vi "MagPhasePlot.vi"(7 "PlotSource":T1, 8 "error in (no error)":errorcluster, 11 "AllData":T3 {"FlukeData"."DataAnalysisArray"."TimeStamp" format="%^<%.3X\n%x>T"; "FlukeData"."ModelDataArray"."FREQUENCY" format="%#_6f"; "FlukeData"."ModelDataArray"."TimeStamp" format="%^<%.3X\n%x>T"; "FlukeData"."PMUDataArray"."FREQUENCY" format="%#_6f"; "FlukeData"."PMUDataArray"."TimeStamp" format="%^<%.3X\n%x>T"; "NISTData"."DataAnlysisArray"."Time" format="%.6f"; "NISTData"."DataAnlysisArray"."TimeStamp" format="%^<%.3X\n%x>T"; "NISTData"."DUTDataArray"."TimeStamp" format="%^<%.3X\n%x>T"; "NISTData"."DUTDataArray"."Time" format="%.6f"; "NISTData"."NIDataArray"."TimeStamp" format="%^<%.3X\n%x>T"; "NISTData"."NIDataArray"."Time" format="%.6f"}) -> (0 "error out":errorcluster, 1 "Phase Plot":T2(graph), 2 "Mag Plot":T2(graph))   [LabVIEW 2014]
uses:
  typedefs/Alldata.ctl
  typedefs/NISTData.ctl
  typedefs/NIDataArray.ctl
  typedefs/NIData.ctl
  typedefs/PhasorRectangular.ctl
  typedefs/DUTData.ctl
  typedefs/NICalcAnalysis.ctl
  typedefs/CalcPhasorError.ctl
  typedefs/PlotDataArrays.ctl
  typedefs/PmuRawDataCluster.ctl
  typedefs/CalcAnalysis.ctl
  typedefs/PlotSource.ctl
  <vilib>/Analysis/coordinate.llb/Angle Units.ctl
  <vilib>/Analysis/coordinate.llb/Angle Range (Degree).ctl
  <vilib>/Analysis/coordinate.llb/Wrap Angle (scalar).vi
  <vilib>/Analysis/NI_AAL_Angle.lvlib
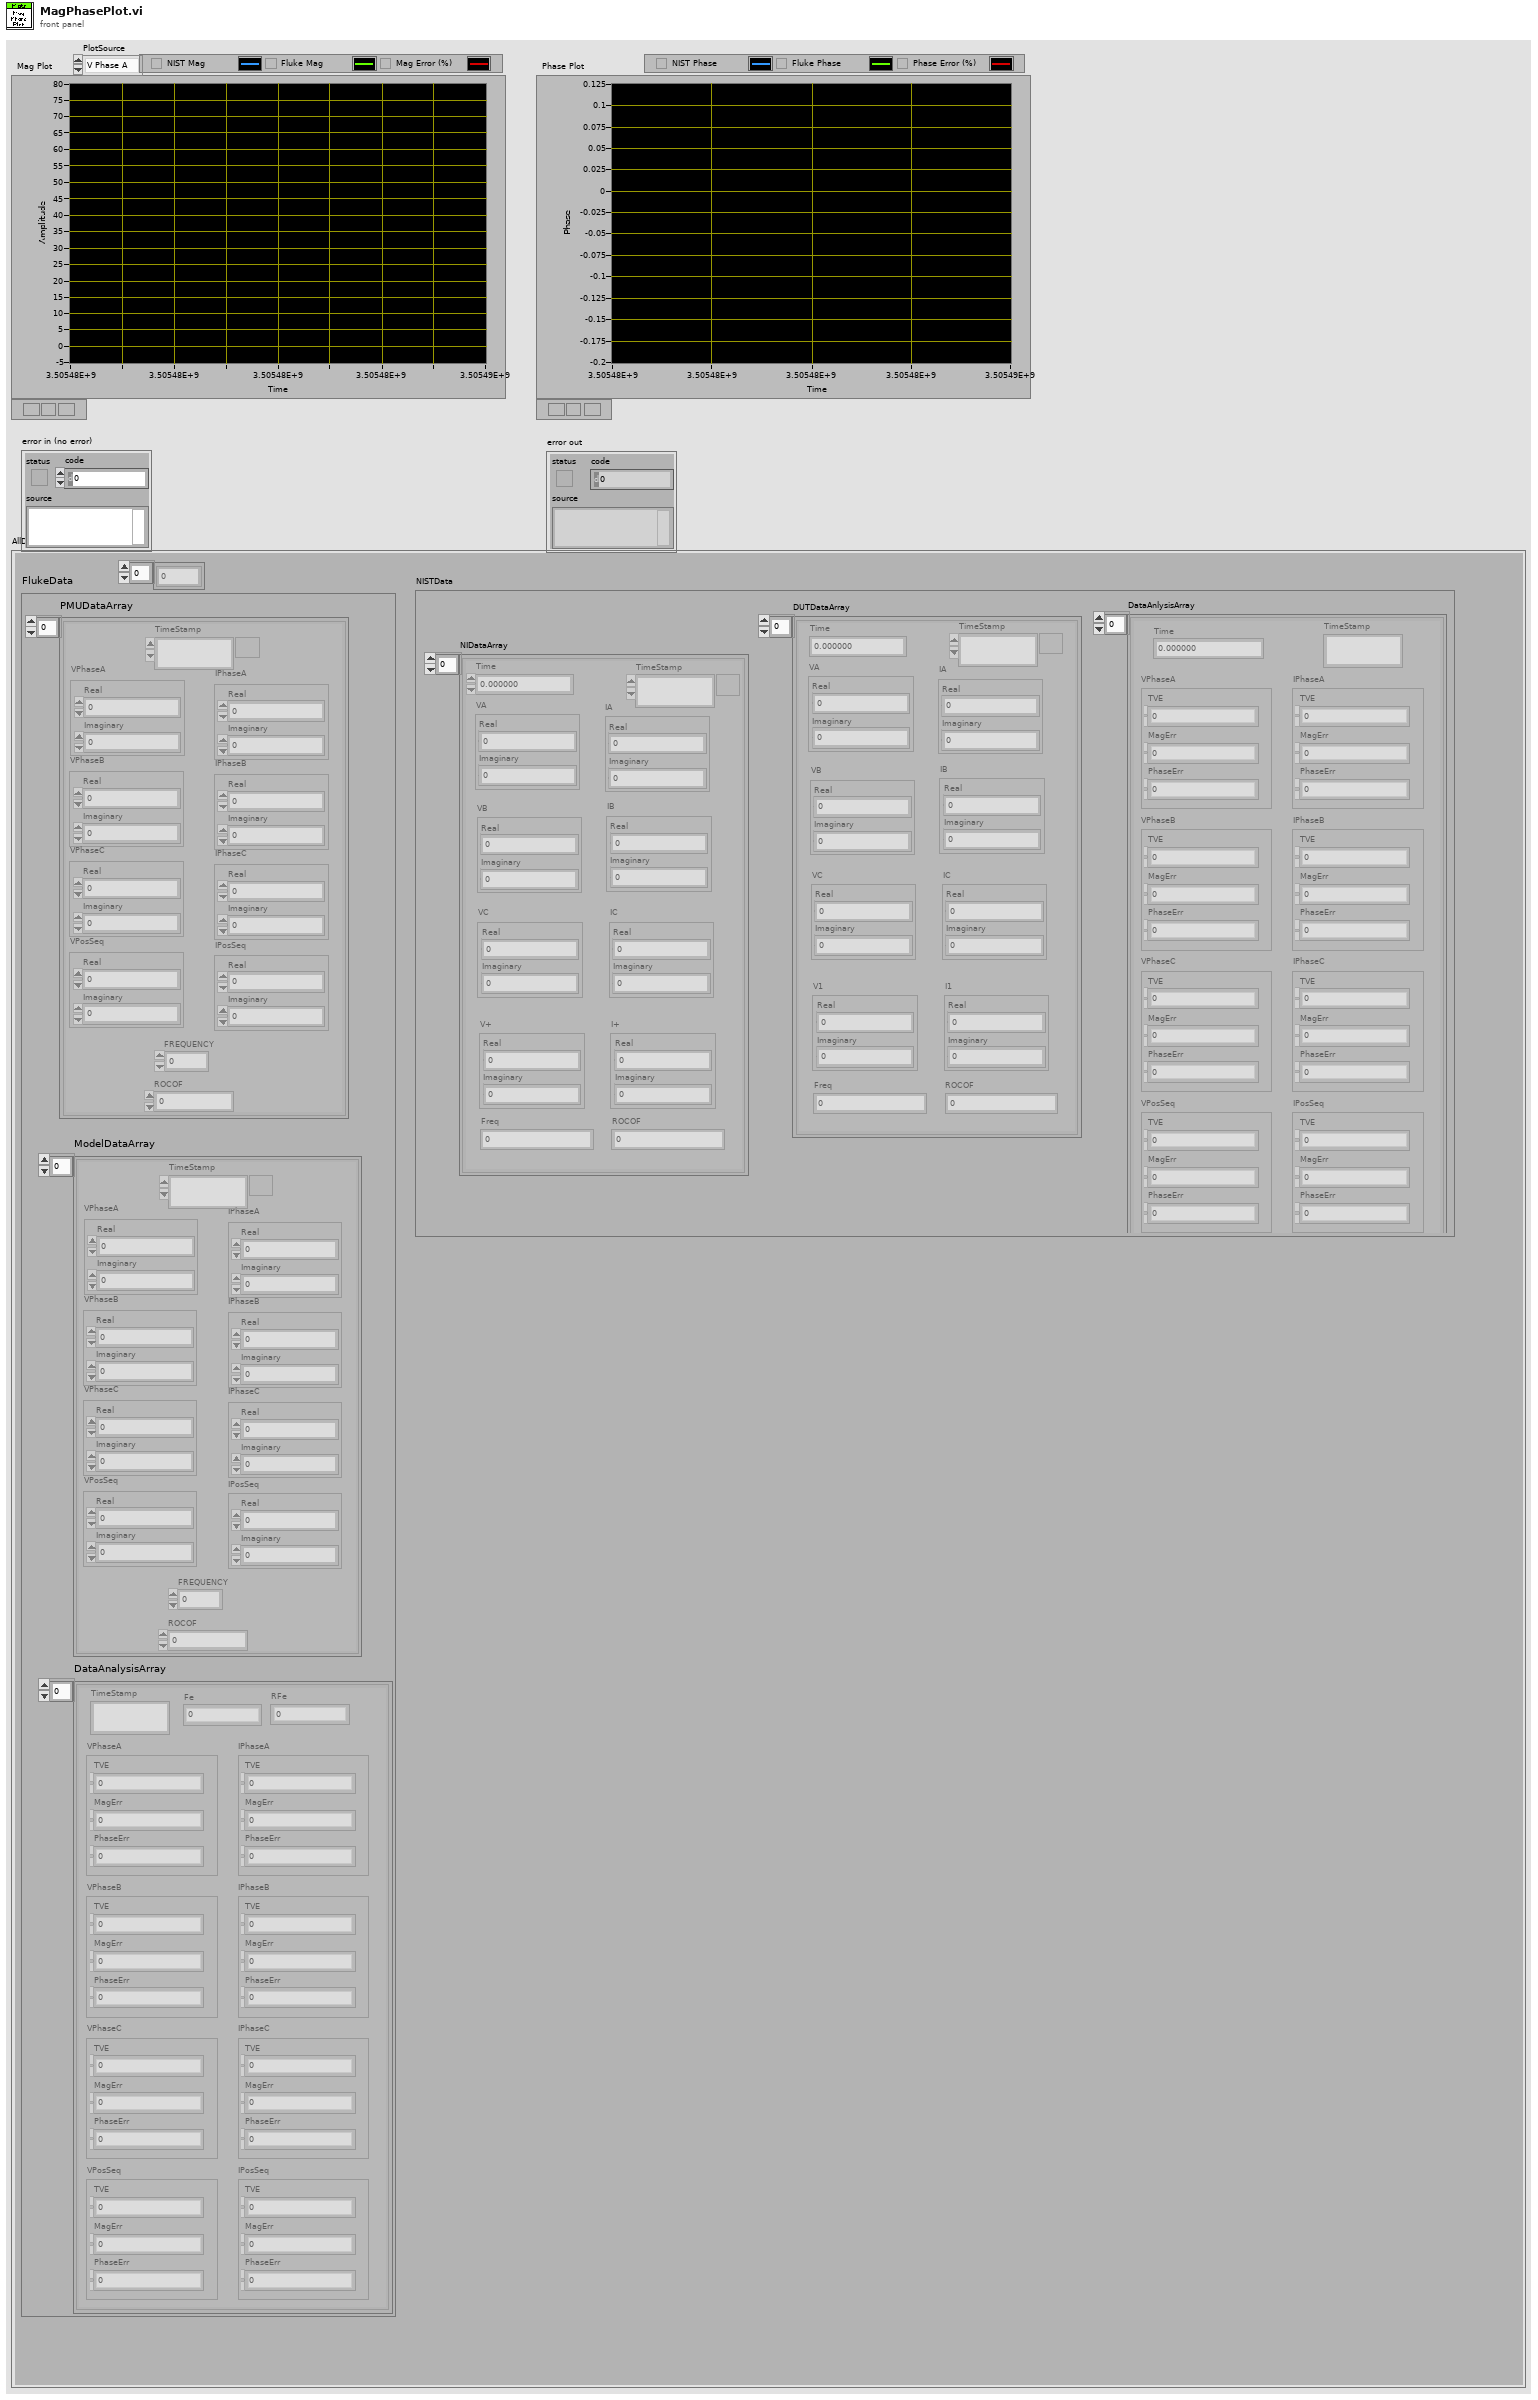
[diagram p1: front panel]
types:
  T1 = typedef "PlotSource.ctl" = enum16{"V Phase A", "V Phase B", "V Phase C", "I Phase A", "I Phase B", "I Phase C"}
  T2 = cluster{"TimestampArray":timestamp[], "Y":dbl[]}[]
  T3 = typedef "Alldata.ctl" = cluster{"NISTData":T4, "FlukeData":T11, "Params":dbl[]}
  T4 = typedef "NISTData.ctl" = cluster{"NIDataArray":T5, "DUTDataArray":T8[], "DataAnlysisArray":T9[]}
  T5 = typedef "NIDataArray.ctl" = T6[]
  T6 = typedef "NIData.ctl" = cluster{"Time":dbl, "VA":T7, "VB":T7, "VC":T7, "V+":T7, "IA":T7, "IB":T7, "IC":T7, "I+":T7, "Freq":dbl, "ROCOF":dbl, "TimeStamp":timestamp}
  T7 = typedef "PhasorRectangular.ctl" = cluster{"Real":dbl, "Imaginary":dbl}
  T8 = typedef "DUTData.ctl" = cluster{"Time":dbl, "VA":T7, "VB":T7, "VC":T7, "V1":T7, "IA":T7, "IB":T7, "IC":T7, "I1":T7, "Freq":dbl, "ROCOF":dbl, "TimeStamp":timestamp}
  T9 = typedef "NICalcAnalysis.ctl" = cluster{"Time":dbl, "VPhaseA":T10, "VPhaseB":T10, "VPhaseC":T10, "VPosSeq":T10, "IPhaseA":T10, "IPhaseB":T10, "IPhaseC":T10, "IPosSeq":T10, "Fe":dbl, "RFe":dbl, "TimeStamp":timestamp}
  T10 = typedef "CalcPhasorError.ctl" = cluster{"TVE":dbl, "MagErr":dbl, "PhaseErr":dbl}
  T11 = typedef "PlotDataArrays.ctl" = cluster{"PMUDataArray":T12[], "ModelDataArray":T12[], "DataAnalysisArray":T13[]}
  T12 = typedef "PmuRawDataCluster.ctl" = cluster{"TimeStamp":timestamp, "VPhaseA":T7, "VPhaseB":T7, "VPhaseC":T7, "VPosSeq":T7, "IPhaseA":T7, "IPhaseB":T7, "IPhaseC":T7, "IPosSeq":T7, "FREQUENCY":dbl, "ROCOF":sgl}
  T13 = typedef "CalcAnalysis.ctl" = cluster{"TimeStamp":timestamp, "VPhaseA":T10, "VPhaseB":T10, "VPhaseC":T10, "VPosSeq":T10, "IPhaseA":T10, "IPhaseB":T10, "IPhaseC":T10, "IPosSeq":T10, "Fe":dbl, "RFe":dbl}
  T14 = typedef "NI_AAL_Angle.lvlib/Angle Units.ctl" = i32
  T15 = typedef "NI_AAL_Angle.lvlib/Angle Range (Degree).ctl" = u16
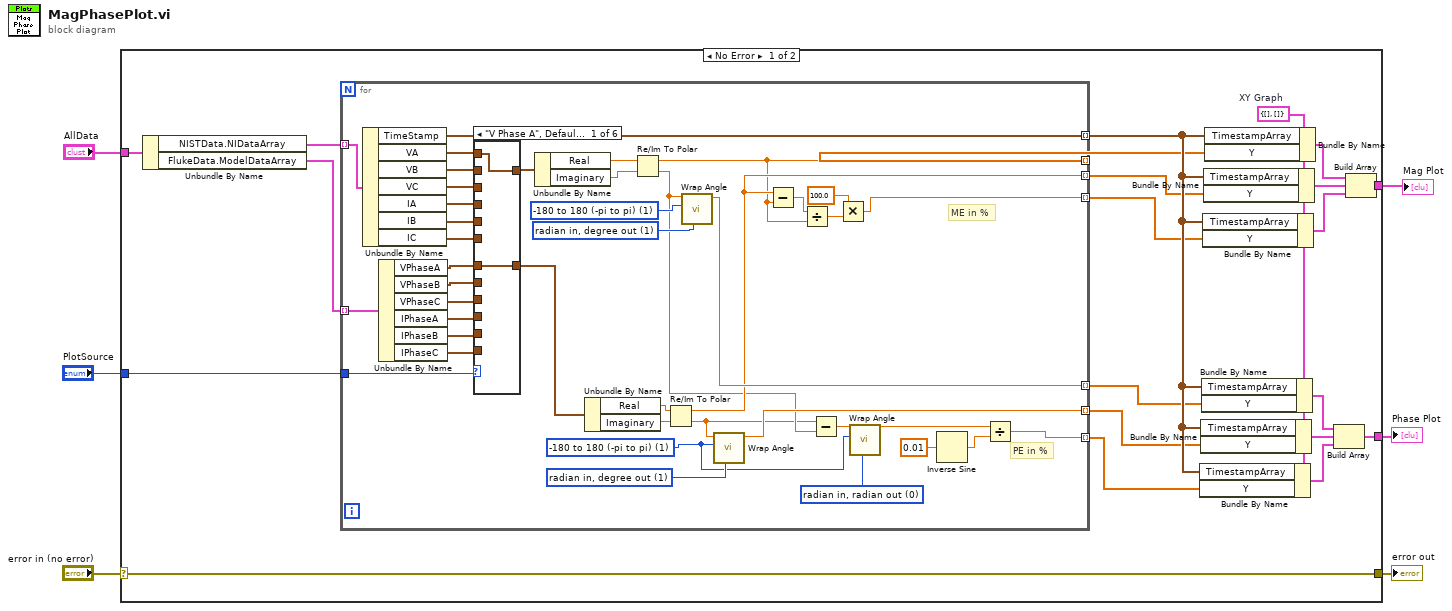
[diagram p0: block diagram]
diagram:
  n1 = case shown="No Error" "error in (no error)" {
    selector: "error in (no error)" -> [w7 w82]
    tunnel: "AllData" -> [w27 _]
    tunnel: [w21 _] -> w5
    tunnel: [w18 _] -> w4
    tunnel: "PlotSource" -> [w14 _]
    tunnel: [w7 w82] -> w1
    frame No Error {
      w17 = cluster{"TimestampArray":timestamp[], "Y":dbl[]} {"TimestampArray"=[], "Y"=[]}  # XY Graph
      n2 = Unbundle By Name(w27) -> ("NISTData.NIDataArray"=w26:T5, "FlukeData.ModelDataArray"=w25:T12[])
      n3 = for {
        tunnel: w26 -> [w69] mode=indexing
        tunnel: [w68] -> w20 mode=indexing
        tunnel: w25 -> [w67] mode=indexing
        tunnel: w14 -> [w66]
        tunnel: [w38] -> w13 mode=indexing
        tunnel: [w40] -> w12 mode=indexing
        tunnel: [w35] -> w11 mode=indexing
        tunnel: [w47] -> w10 mode=indexing
        tunnel: [w48] -> w9 mode=indexing
        tunnel: [w41] -> w8 mode=indexing
        w28 = T14 0 items=["radian in, radian out", "radian in, degree out", "degree in, degree out", "degree in, radian out"] ("angle units")
        w49 = T15 1 items=["none", "-180 to 180 (-pi to pi)", "0 to 360 (0 to 2pi)"] ("angle range")
        w46 = T14 1 items=["radian in, radian out", "radian in, degree out", "degree in, degree out", "degree in, radian out"] ("angle units")
        w29 = T15 1 items=["none", "-180 to 180 (-pi to pi)", "0 to 360 (0 to 2pi)"] ("angle range")
        w30 = T14 1 items=["radian in, radian out", "radian in, degree out", "degree in, degree out", "degree in, radian out"] ("angle units")
        # "ME in %"
        # "PE in %"
        n4 = Unbundle By Name(w69) -> ("TimeStamp"=w68:timestamp, "VA"=w65:T7, "VB"=w64:T7, "VC"=w63:T7, "IA"=w62:T7, "IB"=w61:T7, "IC"=w60:T7)
        n5 = Unbundle By Name(w67) -> ("VPhaseA"=w59:T7, "VPhaseB"=w58:T7, "VPhaseC"=w57:T7, "IPhaseA"=w56:T7, "IPhaseB"=w55:T7, "IPhaseC"=w54:T7)
        n6 = case shown="\"V Phase A\", Default" w66 {
          tunnel: w65 -> [w70 _ _ _ _ _]
          tunnel: w64 -> [_ w73 _ _ _ _]
          tunnel: w63 -> [_ _ w75 _ _ _]
          tunnel: w62 -> [_ _ _ w77 _ _]
          tunnel: w61 -> [_ _ _ _ w79 _]
          tunnel: w60 -> [_ _ _ _ _ w80]
          tunnel: w59 -> [w71 _ _ _ _ _]
          tunnel: w58 -> [_ w72 _ _ _ _]
          tunnel: w57 -> [_ _ w74 _ _ _]
          tunnel: w56 -> [_ _ _ w76 _ _]
          tunnel: w55 -> [_ _ _ _ w78 _]
          tunnel: w54 -> [_ _ _ _ _ w81]
          tunnel: [w70 w73 w75 w77 w79 w80] -> w53
          tunnel: [w71 w72 w74 w76 w78 w81] -> w52
          frame "V Phase A", Default {
          }
          frame "V Phase B" {
          }
          frame "V Phase C" {
          }
          frame "I Phase A" {
          }
          frame "I Phase B" {
          }
          frame "I Phase C" {
          }
        }
        n7 = Unbundle By Name(w53) -> ("Real"=w45:dbl, "Imaginary"=w44:dbl)
        n8 = Unbundle By Name(w52) -> ("Real"=w51:dbl, "Imaginary"=w50:dbl)
        n9 = Re/Im To Polar(2:w44, 3:w45) -> (0:w34:dbl, 1:w38:dbl)
        n10 = Re/Im To Polar(2:w50, 3:w51) -> (0:w33:dbl, 1:w40:dbl)
        n11 = call-poly <vilib>:"Wrap Angle.vi"("angle units"=w46, "angle range"=w49, "angle in"=w34) -> ("angle out"=w47:dbl)  [unwired: 7 in, 1 out]
        n12 = call-poly <vilib>:"Wrap Angle.vi"("angle units"=w30, "angle range"=w29, "angle in"=w33) -> ("angle out"=w48:dbl)  [unwired: 7 in, 1 out]
        n13 = Subtract(x=w40, y=w38) -> (x-y=w39:dbl)
        n14 = Divide(x=w39, y=w38) -> (x/y=w37:dbl)
        n15 = Subtract(x=w33, y=w34) -> (x-y=w32:dbl)
        n16 = Multiply(x=100.0, y=w37) -> (x*y=w35:dbl)
        n17 = call-poly <vilib>:"Wrap Angle.vi"("angle units"=w28, "angle range"=w29, "angle in"=w32) -> ("angle out"=w31:dbl)  [unwired: 7 in, 1 out]
        n18 = Inverse Sine(1:0.01 ("x")) -> (0:w42:dbl)
        n19 = Divide(x=w31, y=w42) -> (x/y=w41:dbl)
      }
      n20 = Bundle By Name(cluster=w17, "TimestampArray"=w20, "Y"=w8) -> (w15:cluster{"TimestampArray":timestamp[], "Y":dbl[]})
      n21 = Bundle By Name(cluster=w17, "TimestampArray"=w20, "Y"=w9) -> (w16:cluster{"TimestampArray":timestamp[], "Y":dbl[]})
      n22 = Bundle By Name(cluster=w17, "TimestampArray"=w20, "Y"=w10) -> (w19:cluster{"TimestampArray":timestamp[], "Y":dbl[]})
      n23 = Bundle By Name(cluster=w17, "TimestampArray"=w20, "Y"=w11) -> (w22:cluster{"TimestampArray":timestamp[], "Y":dbl[]})
      n24 = Bundle By Name(cluster=w17, "TimestampArray"=w20, "Y"=w12) -> (w23:cluster{"TimestampArray":timestamp[], "Y":dbl[]})
      n25 = Bundle By Name(cluster=w17, "TimestampArray"=w20, "Y"=w13) -> (w24:cluster{"TimestampArray":timestamp[], "Y":dbl[]})
      n26 = Build Array(w19, w16, w15) -> (w18:T2)
      n27 = Build Array(w24, w23, w22) -> (w21:T2)
    }
    frame Error {
    }
  }
  "Mag Plot" <- w5
  "Phase Plot" <- w4
  "error out" <- w1
